vi "FTW-Endpoint-Connect.vi"(0 "FTW Endpoint":refnum<class "FTW-Endpoint.lvclass">, 5 "Endpoint Address":T1, 11 "error in":errorcluster) -> (4 "FTW Endpoint out":refnum<class "FTW-Endpoint.lvclass">, 15 "error out":errorcluster)   [LabVIEW 2012, in "FTW-Actor.lvlib" / "FTW-Endpoint.lvclass"]
uses:
  FTW-Endpoint.lvclass
  Utility/FTW-Actor-Address.ctl
  FTW-Endpoint.lvclass/FTW-Endpoint.ctl
  FTW-Actor.lvlib
panel:
  # "Inputs"
  # "Outputs"
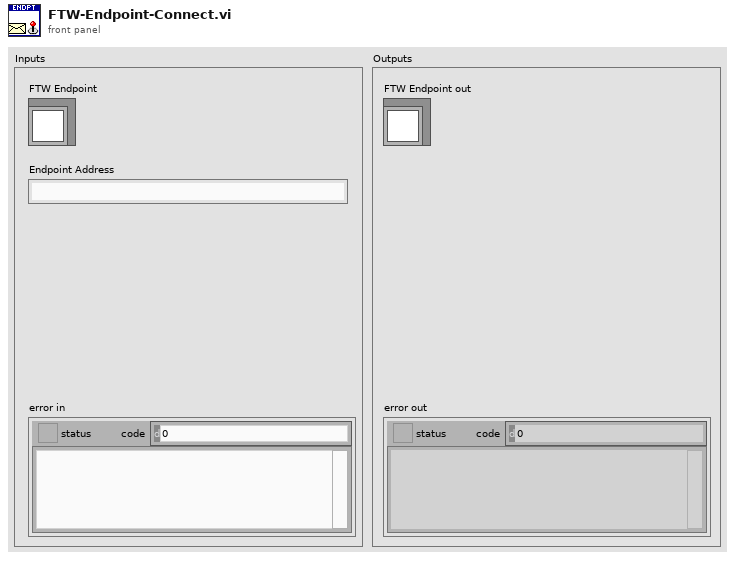
[diagram p1: front panel]
types:
  T1 = typedef "FTW-Actor.lvlib/FTW-Actor-Address.ctl" = string
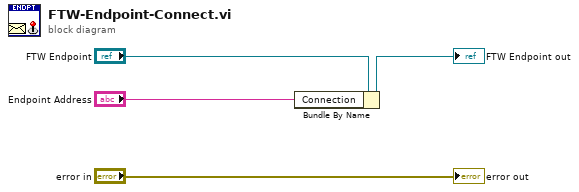
[diagram p0: block diagram]
diagram:
  n1 = Bundle By Name(cluster="FTW Endpoint", "Connection"="Endpoint Address") -> (→"FTW Endpoint out":refnum<class "FTW-Endpoint.lvclass">)
  "error out" <- "error in"
